vi "Initialize.vi"(8 "error in (no error)":errorcluster, 11 "userinfo file":path) -> (0 "error out":errorcluster, 3 "[Data] Userinfo Binary out":refnum<class "[Data] Userinfo Binary.lvclass">)   [LabVIEW 2020, in "[Data] Userinfo Binary.lvclass"]
uses:
  [Data] Userinfo Binary.lvclass
  [Data] Userinfo Binary.lvclass/[Data] Userinfo Binary.ctl
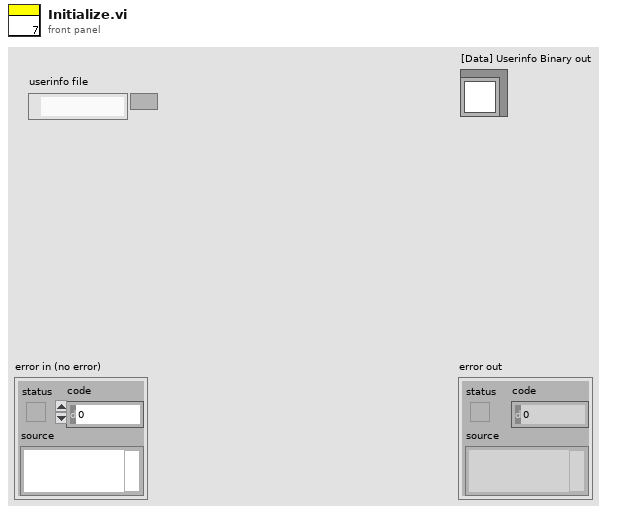
[diagram p1: front panel]
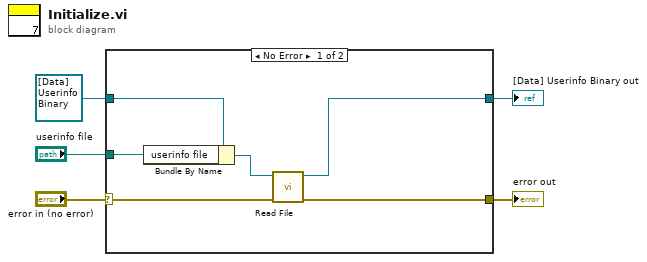
[diagram p0: block diagram]
diagram:
  n1 = case shown="No Error" "error in (no error)" {
    selector: "error in (no error)" -> [w11 w13]
    tunnel: [w6 w13] -> w4
    tunnel: [w7 w12] -> w2
    tunnel: refnum<class "[Data] Userinfo Binary.lvclass"> refnum ("[Data] Userinfo Binary in") -> [w10 w12]
    tunnel: "userinfo file" -> [w9 _]
    frame No Error {
      n2 = Bundle By Name(cluster=w10, "userinfo file"=w9) -> (w8:refnum<class "[Data] Userinfo Binary.lvclass">)
      n3 = call "Read File.vi"("error in (no error)"=w11, "[Data] Userinfo Binary in"=w8) -> ("error out"=w6:errorcluster, "[Data] Userinfo Binary out"=w7:refnum<class "[Data] Userinfo Binary.lvclass">)  [unwired: 8 in]
    }
    frame Error {
    }
  }
  "error out" <- w4
  "[Data] Userinfo Binary out" <- w2
